vi "Items.vi"   [LabVIEW 2020, in "OXYGEN_Datastream.lvlib"]
uses:
  OXYGEN_Datastream.lvlib
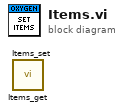
[diagram p0: block diagram]
diagram:
  n1 = call "Items_get.vi"() -> ()  [unwired: 8 in, 4 out]
  n2 = call "Items_set.vi"() -> ()  [unwired: 9 in, 3 out]
